vi "Get Terminal Refs for Unbundle By Name.vi"(8 "error in (no error)":errorcluster, 10 "Unbundler Ref":refnum<vi>, 11 "Getter Generator In":refnum<class "Getter Generator.lvclass">) -> (0 "error out":errorcluster, 2 "reference out":refnum<vi>, 3 "Getter Generator Out":refnum<class "Getter Generator.lvclass">)   [LabVIEW 2020, in "Method Generation.lvlib" / "Getter Generator.lvclass"]
uses:
  Getter Generator.lvclass
  Getter Generator.lvclass/Getter Generator.ctl
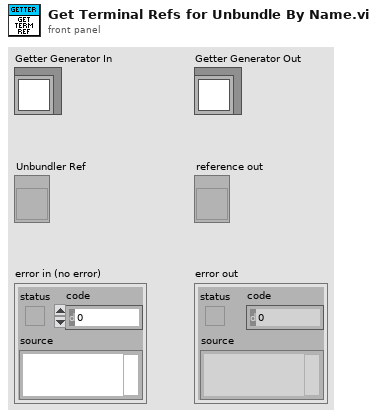
[diagram p1: front panel]
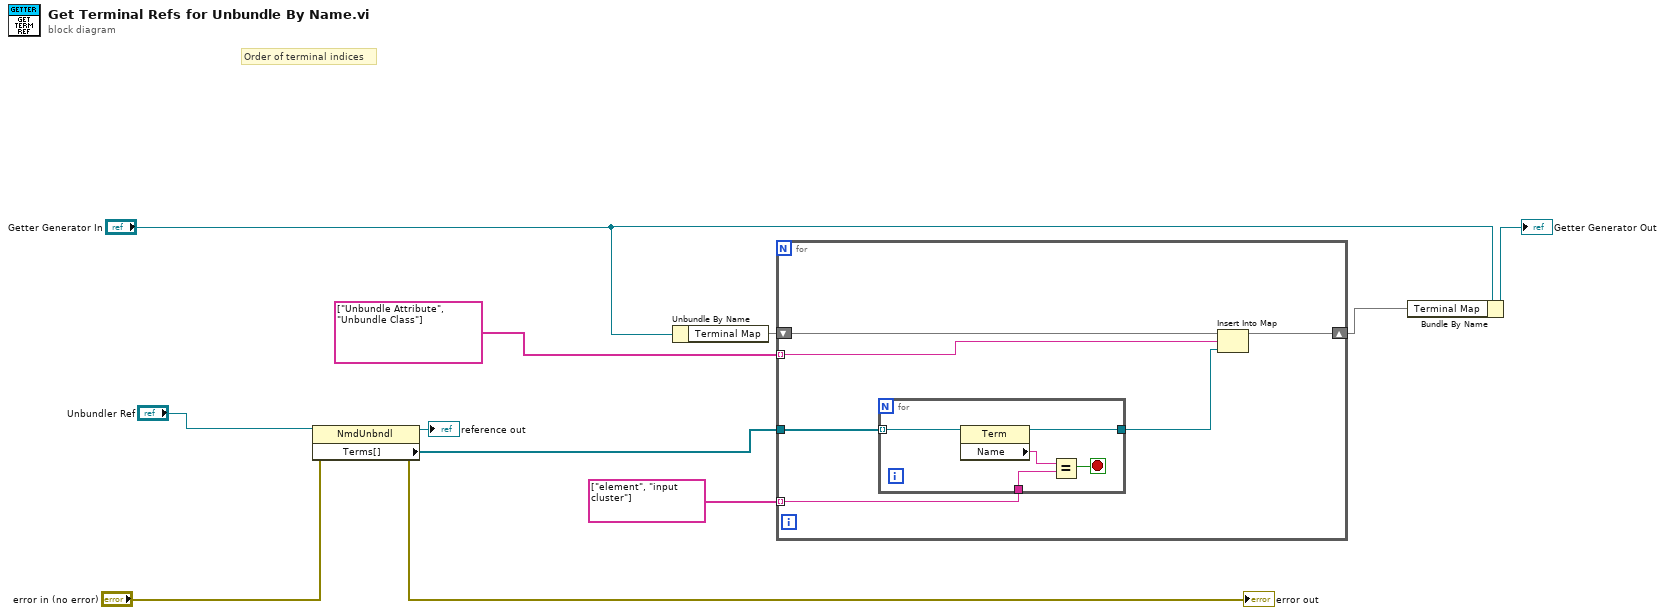
[diagram p0: block diagram]
diagram:
  # "Order of terminal indices"
  n1 = property class="NmdUnbndl"(reference="Unbundler Ref", error in="error in (no error)") -> (reference out=→"reference out":refnum<vi>, error out=→"error out":errorcluster, "Terms[]"=w10:refnum<vi>[])
  n2 = Unbundle By Name("Getter Generator In") -> ("Terminal Map"=w6:map{string, refnum<vi>})
  n3 = for {
    tunnel: w10 -> [w14]
    tunnel: string[] ["Unbundle Attribute", "Unbundle Class"] -> [w16] mode=indexing
    shift-right: [w15] -> w5
    shift-left: w6 -> [w17]
    tunnel: string[] ["element", "input cluster"] -> [w12] mode=indexing
    n4 = for {
      tunnel: w14 -> [w22] mode=indexing
      tunnel: [w21] -> w13
      tunnel: w12 -> [w18]
      stop <- w20 stop-if-true
      n5 = property class="Term"(reference=w22) -> (reference out=w21:refnum<vi>, "Name"=w19:string)  [unwired: 1 in, 1 out]
      n6 = Equal?(x=w19, y=w18) -> (x = y?=w20:bool)
    }
    n7 = Insert Into Map(map in=w17, key=w16, value=w13) -> (map out=w15:map{string, refnum<vi>})  [unwired: 2 out]
  }
  n8 = Bundle By Name(cluster="Getter Generator In", "Terminal Map"=w5) -> (→"Getter Generator Out":refnum<class "Getter Generator.lvclass">)
